vi "Note_to_Freq.vi"(1 "note":i8) -> (0 "frequency":sgl)   [LabVIEW 2009]
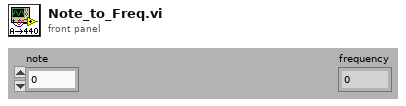
[diagram p1: front panel]
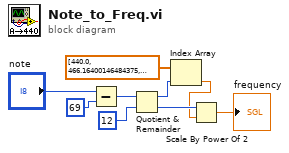
[diagram p0: block diagram]
diagram:
  n1 = Subtract(x="note", y=i8 69) -> (x-y=w4:i8)
  n2 = Quotient & Remainder(x=w4, y=i8 12) -> (x-y*floor(x/y)=w7:i8, floor(x/y)=w9:i8)
  n3 = Index Array(array=sgl[] [440.0, 466.164, 493.883, 523.251, 554.365, 587.33, 622.254, 659.225, 698.456, 739.989, 783.991, 830.609], index=w7) -> (element=w8:sgl)
  n4 = Scale By Power Of 2(n=w9, x=w8) -> (x*2^n=→"frequency":sgl)
